vi "Write Absolute Delay Parameters.vi"(10 "Absolute Delay Parameters":refnum<vi>, 11 "User Interface in":refnum<class "User Interface.lvclass">) -> (3 "User Interface out":refnum<class "User Interface.lvclass">)   [LabVIEW 2016, in "User Interface.lvlib" / "User Interface.lvclass"]
uses:
  User Interface.lvclass
  User Interface.lvclass/User Interface.ctl
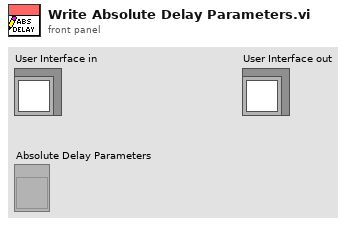
[diagram p1: front panel]
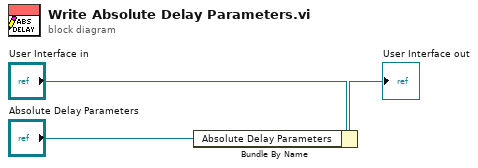
[diagram p0: block diagram]
diagram:
  n1 = Bundle By Name(cluster="User Interface in", "Absolute Delay Parameters"="Absolute Delay Parameters") -> (→"User Interface out":refnum<class "User Interface.lvclass">)
